vi "VI Server Setup.vi"(9 "This VI":refnum<vi>, 10 "This Application":refnum<vi>, 11 "Hello World Event in":refnum<class "Hello World Event.lvclass">) -> (3 "Hello World Event out":refnum<class "Hello World Event.lvclass">)   [LabVIEW 2021, in "Hello World Event.lvlib" / "Hello World Event.lvclass"]
uses:
  Hello World Event.lvclass
  Hello World Event.lvclass/Hello World Event.ctl
  <vilib>/Nathan Davis/jettl/jettl/Event/Event.lvclass
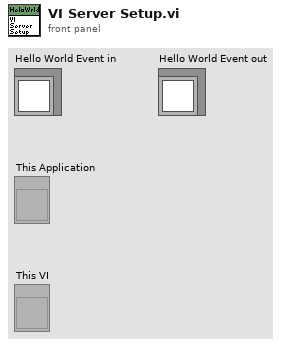
[diagram p1: front panel]
types:
  T1 = enum32{"Invalid", "Standard", "Closed", "Hidden", "Minimized", "Maximized"}
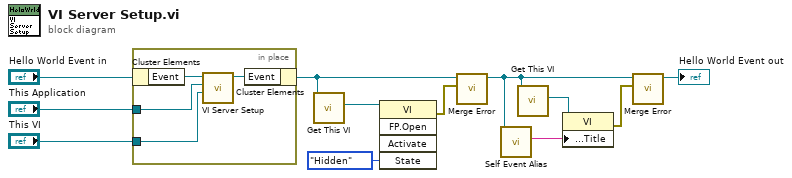
[diagram p0: block diagram]
diagram:
  n1 = in-place {
    in-place-border: "This Application" -> [w14]
    in-place-border: "This VI" -> [w13]
    n2 = in-place-cluster #1("Hello World Event in") -> ("Event"=w16:refnum<class "Event.lvclass">)
    n3 = call-dynamic "VI Server Setup.vi"("This VI"=w13, "This Application"=w14, "jettl in"=w16) -> ("jettl out"=w15:refnum<class "Event.lvclass">)  [unwired: 8 in]
    n4 = in-place-cluster #1("Event"=w15) -> (w1:refnum<class "Hello World Event.lvclass">)
  }
  n5 = call-dynamic "Get This VI.vi"("Hello World Event in"=w1) -> ("This VI"=w7:refnum<vi>)  [unwired: 10 in]
  n6 = invoke class="VI" method="FP.Open"(reference=w7, "State"=T1."Hidden") -> (error out=w5:errorcluster)  [unwired: 3 in, 4 out]
  n7 = call-dynamic "Merge Error.vi"("Error"=w5, "Hello World Event in"=w1) -> ("Hello World Event out"=w3:refnum<class "Hello World Event.lvclass">)  [unwired: 9 in]
  n8 = call-dynamic "Self Event Alias.vi"("Hello World Event in"=w3) -> ("Self Event Alias"=w8:string)  [unwired: 10 in]
  n9 = call-dynamic "Get This VI.vi"("Hello World Event in"=w3) -> ("This VI"=w9:refnum<vi>)  [unwired: 10 in]
  n10 = property class="VI"(reference=w9, "Front Panel.Title"=w8) -> (error out=w4:errorcluster)  [unwired: 1 in, 1 out]
  n11 = call-dynamic "Merge Error.vi"("Error"=w4, "Hello World Event in"=w3) -> ("Hello World Event out"=→"Hello World Event out":refnum<class "Hello World Event.lvclass">)  [unwired: 9 in]
